vi "Undock Display.vi"(8 "error in (no error)":errorcluster, 11 "Assert Display in":refnum<class "Assert Display.lvclass">) -> (0 "error out":errorcluster, 3 "Assert Display out":refnum<class "Assert Display.lvclass">)   [LabVIEW 2016, in "Assert API Components.lvlib" / "Assert Display.lvlib" / "Assert Display.lvclass"]
uses:
  Assert Display.lvclass
  Assert Display.lvclass/Assert Display.ctl
panel:
  out "reference out":refnum<vi>
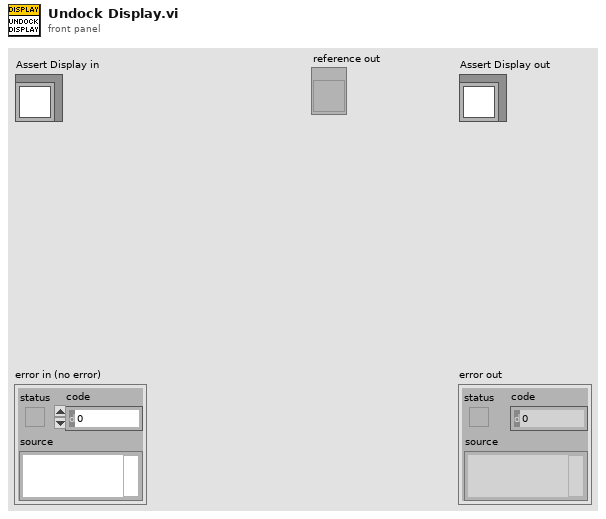
[diagram p1: front panel]
types:
  T1 = enum32{"Invalid", "Standard", "Closed", "Hidden", "Minimized", "Maximized"}
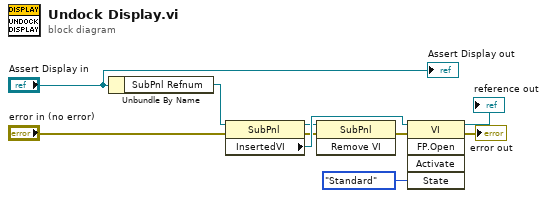
[diagram p0: block diagram]
diagram:
  n1 = Unbundle By Name("Assert Display in") -> ("SubPnl Refnum"=w9:refnum<vi>)
  n2 = property class="SubPnl"(reference=w9, error in="error in (no error)") -> (reference out=w6:refnum<vi>, error out=w5:errorcluster, "InsertedVI"=w8:refnum<vi>)
  n3 = invoke class="SubPnl" method="Remove VI"(reference=w6, error in=w5) -> (error out=w3:errorcluster)  [unwired: 1 in, 2 out]
  n4 = invoke class="VI" method="FP.Open"(reference=w8, error in=w3, "State"=T1."Standard") -> (reference out=→"reference out":refnum<vi>, error out=→"error out":errorcluster)  [unwired: 2 in, 3 out]
  "Assert Display out" <- "Assert Display in"
